vi "Process.vi"(8 "error in":errorcluster, 11 "SMO":refnum<class "SMO.lvclass">) -> (0 "error out":errorcluster, 3 "SMO out":refnum<class "SMO.lvclass">)   [LabVIEW 2013, in "SMO.lvclass"]
uses:
  SMO.lvclass
  Typedefs/Parent Call--Enum.ctl
  Typedefs/SMOState --Enum.ctl
  SMO.lvclass/SMO.ctl
  Support/Attribute.Owner/Packet -- Cluster.ctl
  Support/Attribute/Attribute.lvclass
  Support/Attribute/Attribute.lvclass/Attribute.ctl
  Typedefs/Search Key.ctl
  Private/ReftoDVR--SMO.vi
  <vilib>/Utility/MD5Checksum.llb/MD5Checksum string.vi
  Support/Attribute.Owner/Attribute.Owner.lvclass
panel:
  in  "Test Error":bool
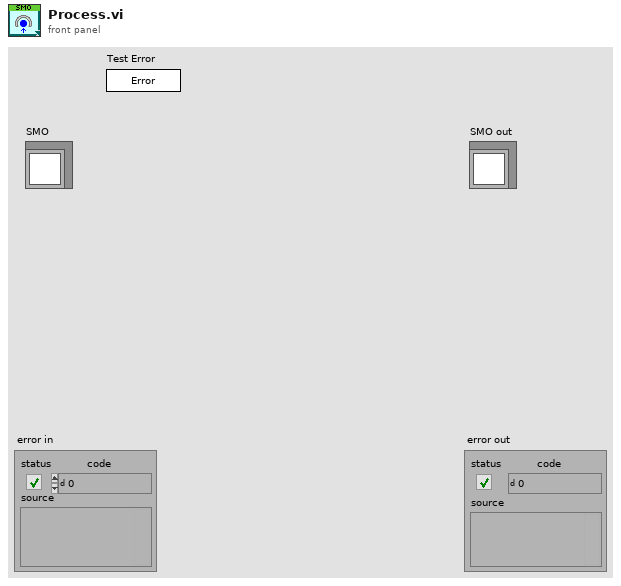
[diagram p1: front panel]
types:
  T1 = typedef "SMO.lvclass/SMOState --Enum.ctl" = enum16{"unknown", "Created", "Started", "Stopped"}
  T2 = typedef "SMO.lvclass/Parent Call--Enum.ctl" = enum16{"Allows parent to run", "Does not request parent to run"}
  T3 = typedef "Attribute.Owner.lvclass/Packet -- Cluster.ctl" = cluster{"Message":string, "Payload":variant, "Source GUID":string}
  T4 = typedef "SMO.lvclass/Search Key.ctl" = enum16{"Name", "GUID", "Qualified Name", "Subsystem Path", "Configuration Path"}
  T5 = typedef "SMO.lvclass/ProcessRegistrationRefnum.ctl" = refnum<event-registration>
  T6 = cluster{"[Dependencies]":refnum<class "SMO.lvclass">[], "State [Dependencies]":refnum<user-event>[], "Error [Dependencies]":refnum<user-event>[], "Message [Dependencies]":refnum<user-event>[]}
  T7 = typedef "def.SMO.lvclass/Scope -- Enum.ctl" = enum16{"Public", "Protected", "Private"}
  T8 = typedef "SMO.lvclass/SMO Dependency Event--Enum.ctl" = enum16{"Added", "Removed", "Started", "Stopped"}
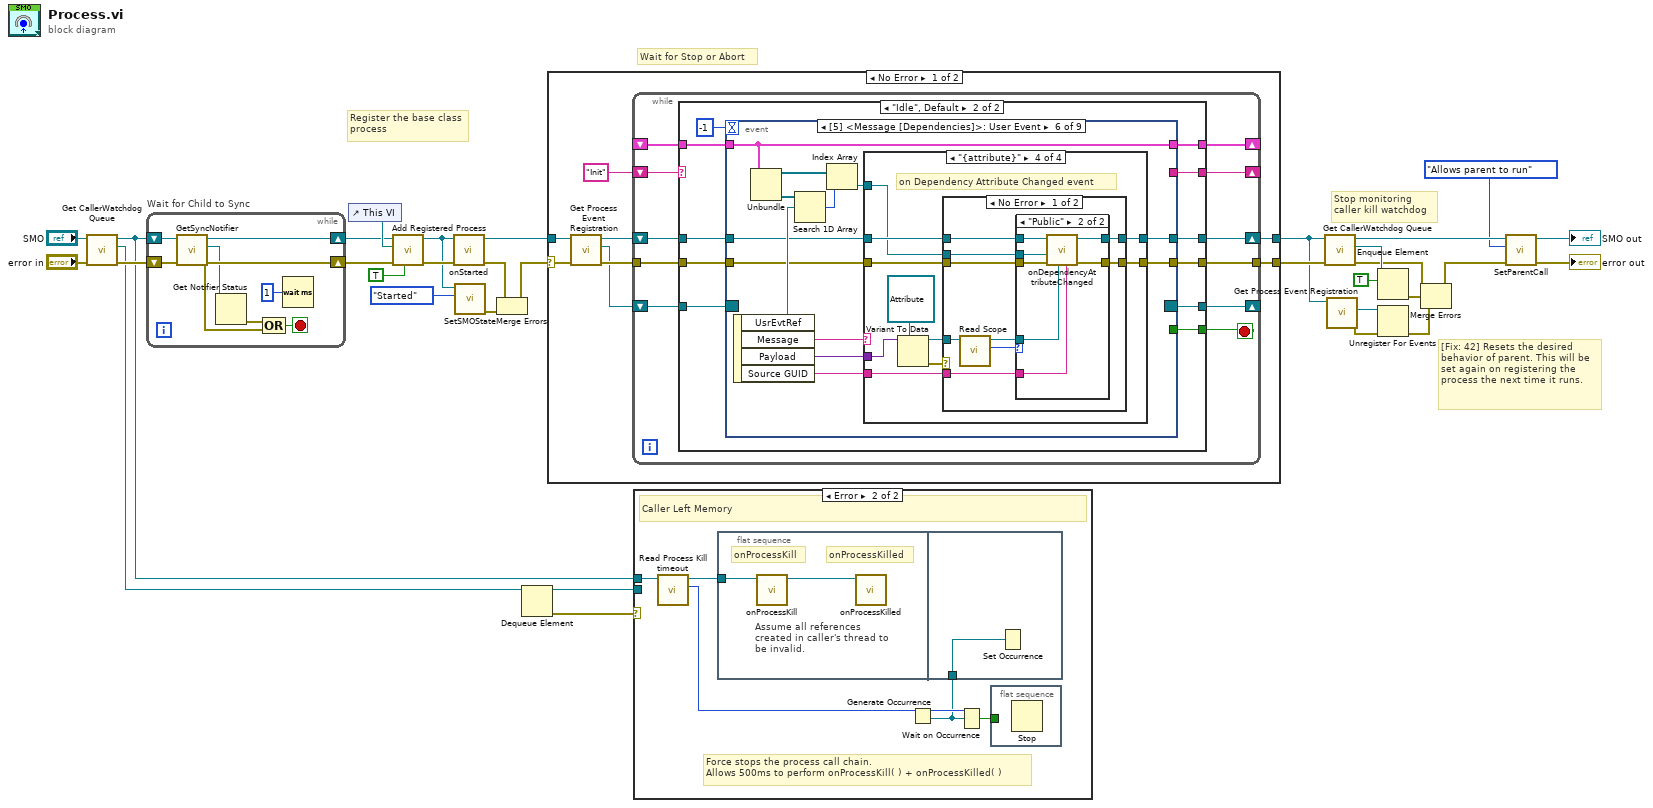
[diagram p0: block diagram]
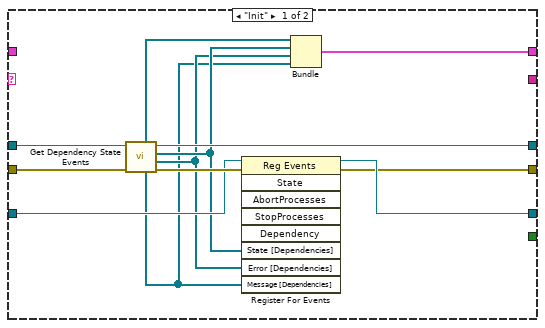
[diagram p3: hidden frame]
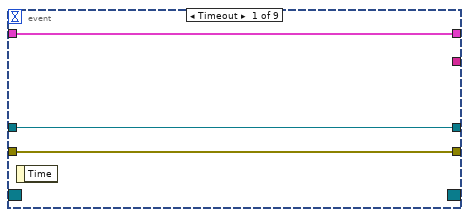
[diagram p4: hidden frame]
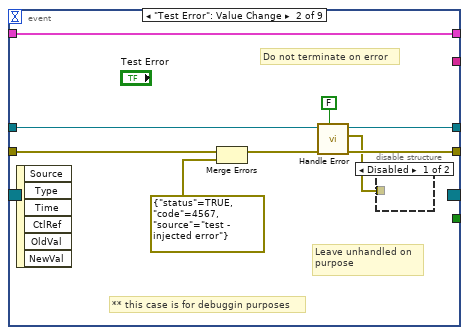
[diagram p5: hidden frame]
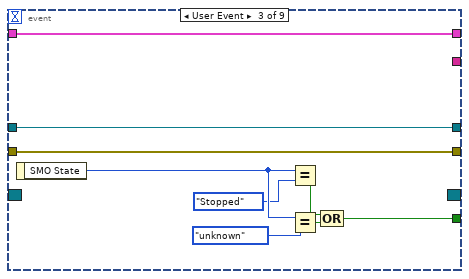
[diagram p7: hidden frame]
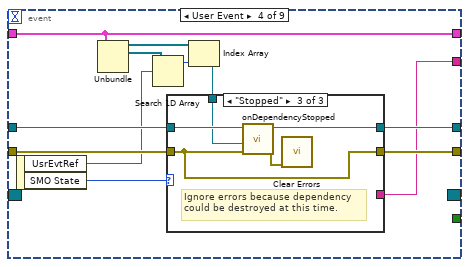
[diagram p8: hidden frame]
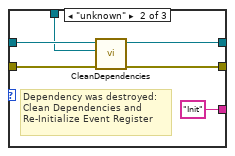
[diagram p10: hidden frame]
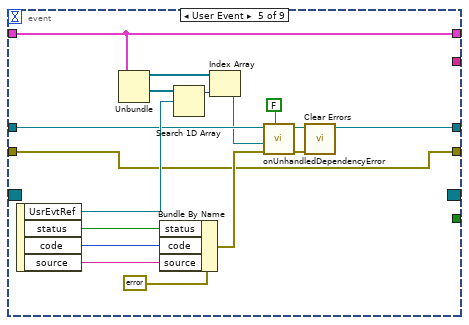
[diagram p11: hidden frame]
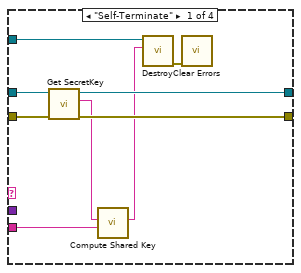
[diagram p12: hidden frame]
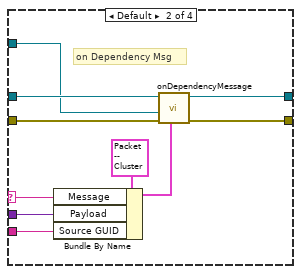
[diagram p13: hidden frame]
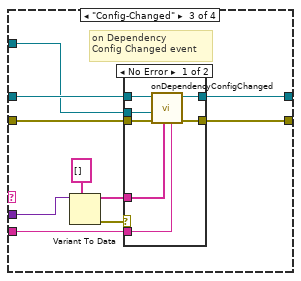
[diagram p14: hidden frame]
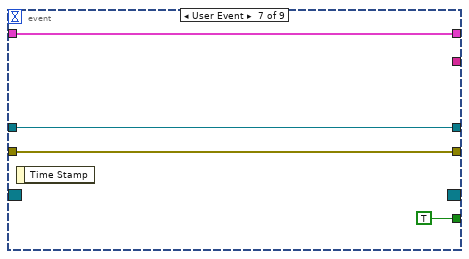
[diagram p18: hidden frame]
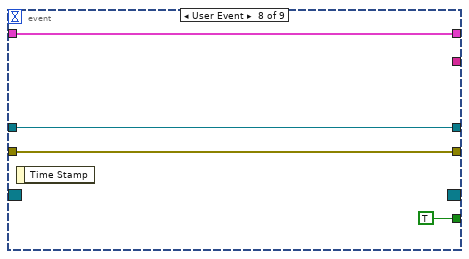
[diagram p19: hidden frame]
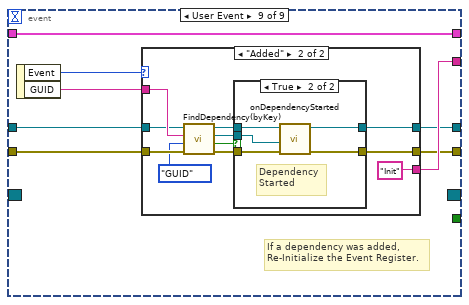
[diagram p20: hidden frame]
diagram:
  # "[Fix: 42] Resets the desired behavior of parent. This will be set again on registering the process the next time it runs."
  # "Stop monitoring\ncaller kill watchdog"
  # "Wait for Stop or Abort"
  # "Register the base class\nprocess"
  n1 = call "Get CallerWatchdog Queue.vi"("error in (no error)"="error in", "SMO in"="SMO") -> ("error out"=w20:errorcluster, "Caller Watchdog"=w19:refnum<queue>, "SMO out"=w18:refnum<class "SMO.lvclass">)  [unwired: 7 in]
  n2 = while "Wait for Child to Sync" {
    shift-right: [w39] -> w11
    shift-left: w18 -> [w40]
    shift-right: [w36] -> w10
    shift-left: w20 -> [w38]
    stop <- w37 stop-if-true
    n3 = call "GetSyncNotifier.vi"("error in (no error)"=w38, "SMO in"=w40) -> ("error out"=w36:errorcluster, "Sync Notifier"=w34:refnum<notifier>, "SMO out"=w39:refnum<class "SMO.lvclass">)  [unwired: 7 in]
    n4 = Get Notifier Status(notifier=w34) -> (error out=w33:errorcluster)  [unwired: 1 in, 4 out]
    n5 = Compound Arithmetic op=OR(w33, w36) -> (w37:bool)
    n6 = Wait (ms)(milliseconds to wait=u32 1) -> ()  [unwired: 1 out]
  }
  n7 = control-ref of="This VI"() -> (w32:refnum<vi>)
  n8 = call "Add Registered Process.vi"("Process Runs (T)"=TRUE, "error in (no error)"=w10, "Process VI (Static VI Ref)"=w32, "SMO"=w11) -> ("error out"=w30:errorcluster, "SMO out"=w8:refnum<class "SMO.lvclass">)  [unwired: 6 in]
  n9 = call-dynamic "onStarted.vi"("error in (no error)"=w30, "SMO"=w8) -> ("error out"=w6:errorcluster, "SMO out"=w17:refnum<class "SMO.lvclass">)  [unwired: 8 in]
  n10 = call "SetSMOState.vi"("SMO State"=SMOState_--Enum."Started" ("event data"), "SMO in"=w8) -> ("error out"=w7:errorcluster)  [unwired: 8 in, 1 out]
  n11 = Merge Errors(w6, w7) -> (w5:errorcluster)
  n12 = Dequeue Element(queue=w19) -> (queue out=w25:refnum<queue>, error out=w26:errorcluster)  [unwired: 2 in, 2 out]
  n13 = case shown="No Error" w5 {
    selector: w5 -> [w44 w264]
    tunnel: [w48 w264] -> w29
    tunnel: w17 -> [w46 w263]
    tunnel: [w47 w263] -> w4
    frame No Error {
      n14 = call "Get Process Event Registration.vi"("error in (no error)"=w44, "SMO in"=w46) -> ("error out"=w43:errorcluster, "Event Registration Refnum"=w42:T5, "SMO out"=w45:refnum<class "SMO.lvclass">)  [unwired: 7 in]
      n15 = while {
        tunnel: [w59] -> w48
        tunnel: w43 -> [w57]
        shift-right: [w52] -> _
        shift-left: "Init" -> [w51]
        shift-right: [w50] -> _
        shift-left: _ -> [w49]
        shift-right: [w56] -> _
        shift-left: w42 -> [w58]
        shift-right: [w54] -> w47
        shift-left: w45 -> [w55]
        stop <- w53 stop-if-true
        n16 = case shown="\"Idle\", Default" w51 {
          tunnel: [w66 w82] -> w59
          tunnel: w58 -> [w68 w81]
          tunnel: w57 -> [w65 w80]
          tunnel: [w67 w79] -> w56
          tunnel: w55 -> [w70 w78]
          tunnel: [w69 w77] -> w54
          tunnel: [_ w75] -> w53
          tunnel: [_ w74] -> w52
          tunnel: [w61 w72] -> w50
          tunnel: w49 -> [_ w73]
          frame "Init" {
            n17 = call "Get Dependency State Events.vi"("error in (no error)"=w65, "SMO in"=w70) -> ("error out"=w71:errorcluster, "Error [Dependencies]"=w62:refnum<user-event>[], "State [Dependencies]"=w63:refnum<user-event>[], "SMO out"=w69:refnum<class "SMO.lvclass">, "Message [Dependencies]"=w60:refnum<user-event>[], "[Dependencies]"=w64:refnum<class "SMO.lvclass">[])  [unwired: 4 in]
            n18 = register-events(reference=w68, error in=w71, w63, w62, w60) -> (reference out=w67:T5, error out=w66:errorcluster)  [unwired: 4 in]
            n19 = Bundle("[Dependencies]"=w64, "State [Dependencies]"=w63, "Error [Dependencies]"=w62, "Message [Dependencies]"=w60) -> (w61:T6)  [unwired: 1 in]
          }
          frame "Idle", Default {
            n20 = event shown="[5] <Message [Dependencies]>: User Event" {
              selector: w81 -> [_ _ _ _ _ _ _ _ _]
              dyn-events: [_ _ _ _ _ _ _ _ _] -> w79
              timeout: -1 -> [_ _ _ _ _ _ _ _ _]
              tunnel: w80 -> [w84 w88 w103 w111 w131 w150 w228 w232 w235]
              tunnel: [w84 w87 w103 w112 w131 w149 w228 w232 w236] -> w82
              tunnel: w78 -> [w85 w92 w99 w114 w135 w152 w229 w233 w238]
              tunnel: [w85 w91 w99 w113 w134 w151 w229 w233 w237] -> w77
              tunnel: [_ _ w96 _ _ _ TRUE TRUE _] -> w75
              tunnel: [_ _ _ w110 _ _ _ _ w239] -> w74
              tunnel: w73 -> [w83 w94 w95 w107 w140 w157 w226 w230 w241]
              tunnel: [w83 w94 w95 w107 w140 w157 w226 w230 w241] -> w72
              event Timeout {
                n21 = event-data() -> ()  [unwired: 1 in, 1 out]
              }
              event "Test Error": Value Change {
                # "** this case is for debuggin purposes"
                # "Leave unhandled on\npurpose"
                # "Do not terminate on error"
                n22 = event-data() -> ()  [unwired: 1 in, 6 out]
                n23 = Merge Errors(w88, errorcluster {"status"=TRUE, "code"=4567, "source"="test - injected error"} ("error in")) -> (w89:errorcluster)
                n24 = call-dynamic "Handle Error.vi"("Stop on Unhandled Error (T)"=FALSE, "error in"=w89, "SMO"=w92) -> ("handling error"=w87:errorcluster, "Unhandled error"=w86:errorcluster, "SMO out"=w91:refnum<class "SMO.lvclass">)  [unwired: 6 in]
                n25 = disable-structure shown="Disabled" {
                  disable-tunnel: w86 -> [_ _]
                  frame Disabled {
                  }
                  frame Enabled {
                  }
                }
              }
              event User Event {
                n26 = event-data() -> ("SMO State"=w98:T1)  [unwired: 1 in]
                n27 = Equal?(x=w98, y=SMOState_--Enum."Stopped") -> (x = y?=w101:bool)
                n28 = Equal?(x=w98, y=SMOState_--Enum."unknown") -> (x = y?=w102:bool)
                n29 = Compound Arithmetic op=OR(w101, w102) -> (w96:bool)
              }
              event User Event {
                n30 = event-data() -> ("UsrEvtRef"=w105:refnum<user-event>, "SMO State"=w115:T1)  [unwired: 1 in]
                n31 = Unbundle(w107) -> ("[Dependencies]"=w108:refnum<class "SMO.lvclass">[], "State [Dependencies]"=w106:refnum<user-event>[])  [unwired: 2 out]
                n32 = Search 1D Array(1D array=w106, element=w105) -> (index of element=w109:i32)  [unwired: 1 in]
                n33 = Index Array(array=w108, index=w109) -> (element=w104:refnum<class "SMO.lvclass">)
                n34 = case shown="\"Stopped\"" w115 {
                  tunnel: w114 -> [w117 w123 w128]
                  tunnel: [w117 w122 w126] -> w113
                  tunnel: [w116 w120 w125] -> w112
                  tunnel: w111 -> [w116 w121 w125]
                  tunnel: [_ "Init" _] -> w110
                  tunnel: w104 -> [_ w118 w127]
                  frame Default {
                  }
                  frame "unknown" {
                    # "Dependency was destroyed:\nClean Dependencies and\nRe-Initialize Event Register"
                    n35 = call "CleanDependencies.vi"("error in (no error)"=w121, "Dependency"=w118, "SMO in"=w123) -> ("error out"=w120:errorcluster, "SMO out"=w122:refnum<class "SMO.lvclass">)  [unwired: 6 in, 1 out]
                  }
                  frame "Stopped" {
                    # "Ignore errors because dependency\ncould be destroyed at this time."
                    n36 = call-dynamic "onDependencyStopped.vi"("error in"=w125, "Dependency"=w127, "SMO in"=w128) -> ("error out"=w124:errorcluster, "SMO out"=w126:refnum<class "SMO.lvclass">)  [unwired: 7 in]
                    n37 = call <vilib>:"Clear Errors.vi"("error in (no error)"=w124) -> ()  [unwired: 6 in, 1 out]
                  }
                }
              }
              event User Event {
                n38 = event-data() -> ("UsrEvtRef"=w138:refnum<user-event>, "status"=w141:bool, "code"=w142:i32, "source"=w143:string)  [unwired: 1 in]
                n39 = Unbundle(w140) -> ("[Dependencies]"=w137:refnum<class "SMO.lvclass">[], "Error [Dependencies]"=w139:refnum<user-event>[])  [unwired: 2 out]
                n40 = Bundle By Name(cluster=errorcluster {"status"=FALSE, "code"=0, "source"=""} ("error constant"), "status"=w141, "code"=w142, "source"=w143) -> (w133:errorcluster)
                n41 = Search 1D Array(1D array=w139, element=w138) -> (index of element=w136:i32)  [unwired: 1 in]
                n42 = Index Array(array=w137, index=w136) -> (element=w132:refnum<class "SMO.lvclass">)
                n43 = call-dynamic "onUnhandledDependencyError.vi"("Stop on Unhandled Error (F)"=FALSE, "Unhandled Dependency Error"=w133, "Dependency"=w132, "SMO in"=w135) -> ("Unhandled error"=w129:errorcluster, "SMO out"=w134:refnum<class "SMO.lvclass">)  [unwired: 6 in]
                n44 = call <vilib>:"Clear Errors.vi"("error in (no error)"=w129) -> ()  [unwired: 6 in, 1 out]
              }
              event User Event {
                n45 = event-data() -> ("UsrEvtRef"=w156:refnum<user-event>, "Message"=w153:string, "Payload"=w146:variant, "Source GUID"=w147:string)  [unwired: 1 in]
                n46 = Unbundle(w157) -> ("[Dependencies]"=w155:refnum<class "SMO.lvclass">[], "Message [Dependencies]"=w154:refnum<user-event>[])  [unwired: 2 out]
                n47 = Search 1D Array(1D array=w154, element=w156) -> (index of element=w145:i32)  [unwired: 1 in]
                n48 = Index Array(array=w155, index=w145) -> (element=w148:refnum<class "SMO.lvclass">)
                n49 = case shown="\"{attribute}\"" w153 {
                  selector: w153 -> [_ w169 _ _]
                  tunnel: w152 -> [w166 w176 w186 w205]
                  tunnel: [w165 w175 w185 w204] -> w151
                  tunnel: w150 -> [w164 w174 w184 w203]
                  tunnel: [w163 w173 w182 w201] -> w149
                  tunnel: w148 -> [w161 w172 w183 w202]
                  tunnel: w147 -> [w162 w167 w181 w200]
                  tunnel: w146 -> [_ w168 w180 w199]
                  frame "Self-Terminate" {
                    n50 = call "Get SecretKey.vi"("error in (no error)"=w164, "SMO"=w166) -> ("error out"=w163:errorcluster, "SecretKey"=w158:string, "SMO out"=w165:refnum<class "SMO.lvclass">)  [unwired: 7 in]
                    n51 = call "Compute Shared Key.vi"("GUID"=w162, "SecretKey"=w158) -> ("Shared Key"=w160:string)  [unwired: 9 in]
                    n52 = call "Destroy.vi"("Shared Key"=w160, "SMO"=w161) -> ("error out"=w159:errorcluster)  [unwired: 9 in]
                    n53 = call <vilib>:"Clear Errors.vi"("error in (no error)"=w159) -> ()  [unwired: 6 in, 1 out]
                  }
                  frame Default {
                    # "on Dependency Msg"
                    n54 = Bundle By Name(cluster=T3 {"Message"="", "Payload"=variant, "Source GUID"=""} ("Packet"), "Message"=w169, "Payload"=w168, "Source GUID"=w167) -> (w171:T3)
                    n55 = call-dynamic "onDependencyMessage.vi"("Packet"=w171, "error in"=w174, "Dependency"=w172, "SMO in"=w176) -> ("error out"=w173:errorcluster, "SMO out"=w175:refnum<class "SMO.lvclass">)  [unwired: 6 in]
                  }
                  frame "Config-Changed" {
                    # "on Dependency\nConfig Changed event"
                    n56 = Variant To Data(type=string[] [] ("keys changed"), Variant=w180) -> (data=w178:string[], error out=w177:errorcluster)  [unwired: 1 in]
                    n57 = case shown="No Error" w177 {
                      tunnel: w186 -> [w193 w195]
                      tunnel: [w192 w195] -> w185
                      tunnel: w184 -> [w191 w194]
                      tunnel: w183 -> [w190 _]
                      tunnel: [w189 w194] -> w182
                      tunnel: w181 -> [w188 _]
                      tunnel: w178 -> [w187 _]
                      frame No Error {
                        n58 = call-dynamic "onDependencyConfigChanged.vi"("Source GUID"=w188, "keys changed"=w187, "error in"=w191, "Dependency"=w190, "SMO in"=w193) -> ("error out"=w189:errorcluster, "SMO out"=w192:refnum<class "SMO.lvclass">)  [unwired: 5 in]
                      }
                      frame Error {
                      }
                    }
                  }
                  frame "{attribute}" {
                    # "on Dependency Attribute Changed event"
                    n59 = Variant To Data(type=refnum<class "Attribute.lvclass"> refnum ("Attribute"), Variant=w199) -> (data=w198:refnum<class "Attribute.lvclass">, error out=w197:errorcluster)  [unwired: 1 in]
                    n60 = case shown="No Error" w197 {
                      tunnel: w205 -> [w214 w225]
                      tunnel: [w213 w225] -> w204
                      tunnel: w203 -> [w211 w224]
                      tunnel: w202 -> [w210 _]
                      tunnel: [w212 w224] -> w201
                      tunnel: w200 -> [w209 _]
                      tunnel: w198 -> [w208 _]
                      frame No Error {
                        n61 = call "Read Scope.vi"("Attribute in"=w208) -> ("Scope"=w206:T7, "Attribute out"=w207:refnum<class "Attribute.lvclass">)  [unwired: 9 in]
                        n62 = case shown="\"Public\"" w206 {
                          tunnel: w214 -> [w216 w223]
                          tunnel: [w216 w222] -> w213
                          tunnel: [w215 w221] -> w212
                          tunnel: w211 -> [w215 w220]
                          tunnel: w210 -> [_ w219]
                          tunnel: w209 -> [_ w218]
                          tunnel: w207 -> [_ w217]
                          frame Default {
                          }
                          frame "Public" {
                            n63 = call-dynamic "onDependencyAttributeChanged.vi"("Source GUID"=w218, "Attribute"=w217, "error in"=w220, "Dependency"=w219, "SMO in"=w223) -> ("error out"=w221:errorcluster, "SMO out"=w222:refnum<class "SMO.lvclass">)  [unwired: 5 in]
                          }
                        }
                      }
                      frame Error {
                      }
                    }
                  }
                }
              }
              event User Event {
                n64 = event-data() -> ()  [unwired: 1 in, 1 out]
              }
              event User Event {
                n65 = event-data() -> ()  [unwired: 1 in, 1 out]
              }
              event User Event {
                # "If a dependency was added,\nRe-Initialize the Event Register."
                n66 = event-data() -> ("Event"=w240:T8, "GUID"=w234:string)  [unwired: 1 in]
                n67 = case shown="\"Added\"" w240 {
                  tunnel: ["Idle" "Init"] -> w239
                  tunnel: w238 -> [w243 w253]
                  tunnel: [w243 w247] -> w237
                  tunnel: [w242 w246] -> w236
                  tunnel: w235 -> [w242 w252]
                  tunnel: w234 -> [_ w254]
                  frame Default {
                  }
                  frame "Added" {
                    n68 = call "FindDependency(byKey).vi"("error in (no error)"=w252, "Search Key (Name)"=Search_Key."GUID", "Key"=w254, "SMO in"=w253) -> ("error out"=w249:errorcluster, "Found?"=w250:bool, "Dependency"=w245:refnum<class "SMO.lvclass">, "SMO dup"=w248:refnum<class "SMO.lvclass">)  [unwired: 4 in]
                    n69 = case shown="True" w250 {
                      tunnel: w249 -> [w256 w259]
                      tunnel: w248 -> [w257 w262]
                      tunnel: [w257 w260] -> w247
                      tunnel: [w256 w258] -> w246
                      tunnel: w245 -> [_ w261]
                      frame False {
                      }
                      frame True {
                        # "Dependency\nStarted"
                        n70 = call-dynamic "onDependencyStarted.vi"("error in"=w259, "Dependency"=w261, "SMO in"=w262) -> ("error out"=w258:errorcluster, "SMO out"=w260:refnum<class "SMO.lvclass">)  [unwired: 7 in]
                      }
                    }
                  }
                }
              }
            }
          }
        }
      }
    }
    frame Error {
    }
  }
  n71 = case shown="Error" w26 {
    tunnel: w25 -> [_ _]
    tunnel: w18 -> [_ w268]
    frame No Error {
      # "Process Terminated Normally"
    }
    frame Error {
      # "Force stops the process call chain.\nAllows 500ms to perform onProcessKill( ) + onProcessKilled( )"
      # "Caller Left Memory"
      n72 = call "Read Process Kill timeout.vi"("SMO in"=w268) -> ("Process Kill timeout (ms)"=w266:i32, "SMO out"=w267:refnum<class "SMO.lvclass">)  [unwired: 9 in]
      n73 = flat-sequence {
        tunnel: w267 -> [w271]
        tunnel: w265 -> [w272]
        frame #0 {
          # "Assume all references created in caller's thread to be invalid."
          # "onProcessKilled"
          # "onProcessKill"
          n74 = call-dynamic "onProcessKill.vi"("SMO in"=w271) -> ("SMO out"=w270:refnum<class "SMO.lvclass">)  [unwired: 10 in]
          n75 = call-dynamic "onProcessKilled.vi"("SMO in"=w270) -> ()  [unwired: 11 in]
        }
        frame #1 {
          n76 = Set Occurrence(w272) -> ()
        }
      }
      n77 = Generate Occurrence() -> (w265:refnum<k4>)
      n78 = Wait on Occurrence(2:w265, 3:w266) -> (0:w269:bool)  [unwired: 1 in]
      n79 = flat-sequence {
        tunnel: w269 -> [_]
        frame #0 {
          n80 = Stop() -> ()  [unwired: 1 in]
        }
      }
    }
  }
  n81 = call "Get CallerWatchdog Queue.vi"("error in (no error)"=w29, "SMO in"=w4) -> ("error out"=w23:errorcluster, "Caller Watchdog"=w28:refnum<queue>, "SMO out"=w14:refnum<class "SMO.lvclass">)  [unwired: 7 in]
  n82 = call "Get Process Event Registration.vi"("SMO in"=w4) -> ("error out"=w1:errorcluster, "Event Registration Refnum"=w3:T5)  [unwired: 8 in, 1 out]
  n83 = Enqueue Element(queue=w28, element=TRUE) -> (error out=w24:errorcluster)  [unwired: 2 in, 2 out]
  n84 = Unregister For Events(event registration refnum=w3, error in=w1) -> (error out=w2:errorcluster)
  n85 = Merge Errors(w23, w24, w2) -> (w16:errorcluster)
  n86 = call "SetParentCall.vi"("error in (no error)"=w16, "Parent Call"=Parent_Call--Enum."Allows parent to run", "SMO in"=w14) -> ("error out"=→"error out":errorcluster, "SMO out"=→"SMO out":refnum<class "SMO.lvclass">)  [unwired: 7 in]
